vi "Read Recovery File.vi"(8 "error in (no error)":errorcluster, 11 "Path":path) -> (0 "error out":errorcluster, 2 "Data Out":dbl[](array[numeric]))   [LabVIEW 2022 SP3]
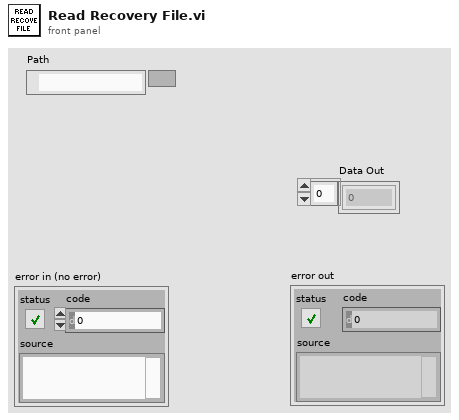
[diagram p1: front panel]
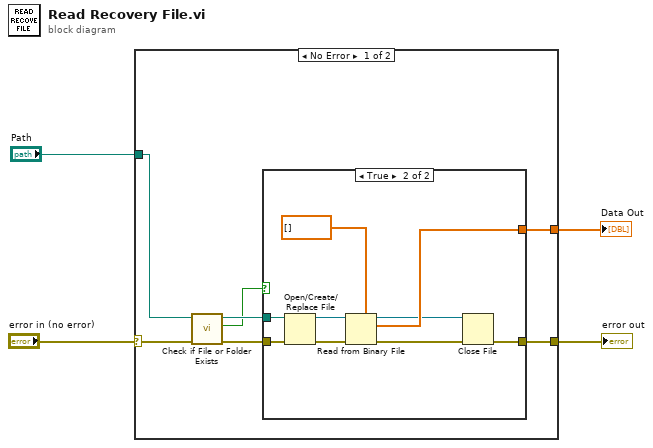
[diagram p0: block diagram]
diagram:
  n1 = case shown="No Error" "error in (no error)" {
    selector: "error in (no error)" -> [w9 w22]
    tunnel: [w11 w22] -> w3
    tunnel: "Path" -> [w7 _]
    tunnel: [w10 _] -> w1
    frame No Error {
      n2 = call <vilib>:"Check if File or Folder Exists.vi"("error in (no error)"=w9, "path"=w7) -> ("error out"=w8:errorcluster, "file or folder exists?"=w5:bool, "dup path"=w6:path)  [unwired: 7 in]
      n3 = case shown="True" w5 {
        tunnel: [w12 w21] -> w11
        tunnel: [_ w17] -> w10
        tunnel: w8 -> [w12 w14]
        tunnel: w6 -> [_ w13]
        frame False {
        }
        frame True {
          n4 = Open/Create/Replace File(file path (use dialog)=w13, error in=w14) -> (refnum out=w15:refnum<file>, error out=w20:errorcluster)  [unwired: 4 in, 1 out]
          n5 = Read from Binary File(5:dbl[] [], 8:w20, 11:w15) -> (0:w19:errorcluster, 2:w17:dbl[], 3:w16:refnum<file>)  [unwired: 3 in, 1 out]
          n6 = Close File(refnum=w16, error in=w19) -> (error out=w21:errorcluster)  [unwired: 1 out]
        }
      }
    }
    frame Error {
    }
  }
  "error out" <- w3
  "Data Out" <- w1
